vi "Read wait multiplier.vi"(8 "error in (no error)":errorcluster, 11 "RTU Data Unit in":refnum<class "RTU Data Unit.lvclass">) -> (0 "error out":errorcluster, 2 "wait multiplier":sgl, 3 "RTU Data Unit out":refnum<class "RTU Data Unit.lvclass">)   [LabVIEW 2021, in "RTU Data Unit.lvclass"]
uses:
  RTU Data Unit.lvclass
  RTU Data Unit.lvclass/RTU Data Unit.ctl
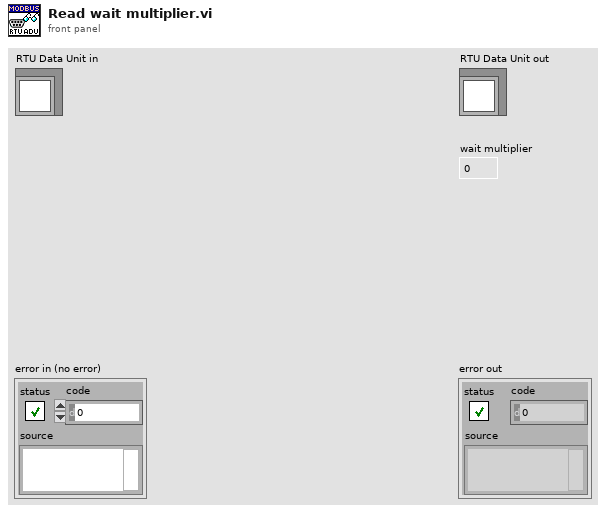
[diagram p1: front panel]
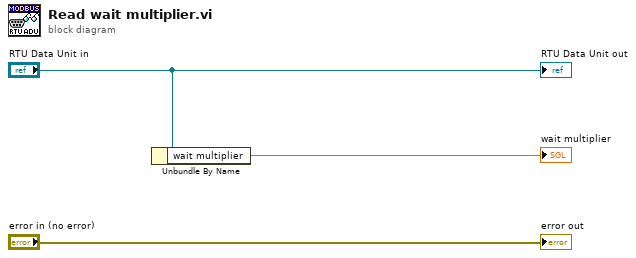
[diagram p0: block diagram]
diagram:
  n1 = Unbundle By Name("RTU Data Unit in") -> ("wait multiplier"=→"wait multiplier":sgl)
  "error out" <- "error in (no error)"
  "RTU Data Unit out" <- "RTU Data Unit in"
